vi "Get Injected Value.vi"(8 "error in (no error)":errorcluster, 11 "Fault-Injection_Boolean_Type in":refnum<class "Fault-Injection_U8_Type.lvclass">) -> (0 "error out":errorcluster, 2 "Value":u8, 3 "Fault-Injection_Boolean_Type out":refnum<class "Fault-Injection_U8_Type.lvclass">)   [LabVIEW 2021, in "Fault-Injection_U8_Type.lvclass"]
uses:
  Fault-Injection_U8_Type.lvclass
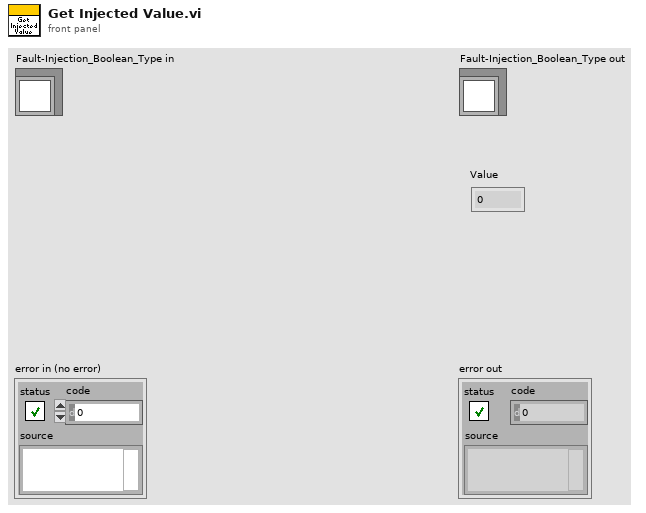
[diagram p1: front panel]
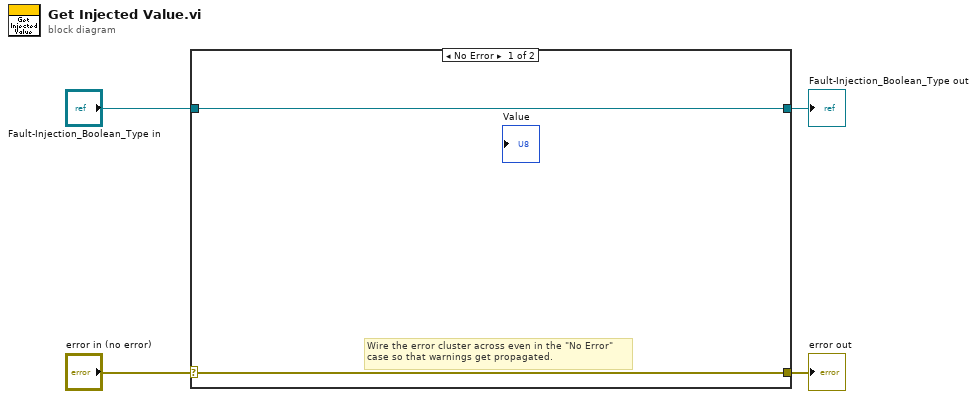
[diagram p0: block diagram]
diagram:
  n1 = case shown="No Error" "error in (no error)" {
    selector: "error in (no error)" -> [w5 w8]
    tunnel: [w5 w8] -> w3
    tunnel: [w6 w7] -> w1
    tunnel: "Fault-Injection_Boolean_Type in" -> [w6 w7]
    frame No Error {
      # "Wire the error cluster across even in the \"No Error\"\ncase so that warnings get propagated."
    }
    frame Error {
    }
  }
  "error out" <- w3
  "Fault-Injection_Boolean_Type out" <- w1
